vi "mainOcto_Scanning.vi"() -> ()   [LabVIEW 2013]
uses:
  <userlib>/Octoplus_LIDAR/GlobalNameAngles.vi
  <userlib>/Octoplus_LIDAR/Octoplus_LIDAR.lvlib
  <vilib>/Analysis/NI_AALBase.lvlib
panel:
  in  "start scan":bool
  in  "VISA resource name":refnum<visa-resource-name>
  in  "Time (ms)":u32
  in  "Azh":u16[](array[numeric])
  in  "Alt":u16[](array[numeric])
  in  "Nbr of lines in Image":u32=6000
  in  "File Path":path=path "D:/Sat25"
  in  "Capture":bool
  in  "Record data":bool
  in  "Timeslot (cw, ts1, ts2)":i32(knob)=2 scale=0.0..2.0
  out "Background":dbl[](graph)
  in  "start":bool
  out "Signal":dbl[][](graph)
  out "iteration":i32
  in  "stop":bool
  in  "error in (no error)":errorcluster
  out "error out":errorcluster
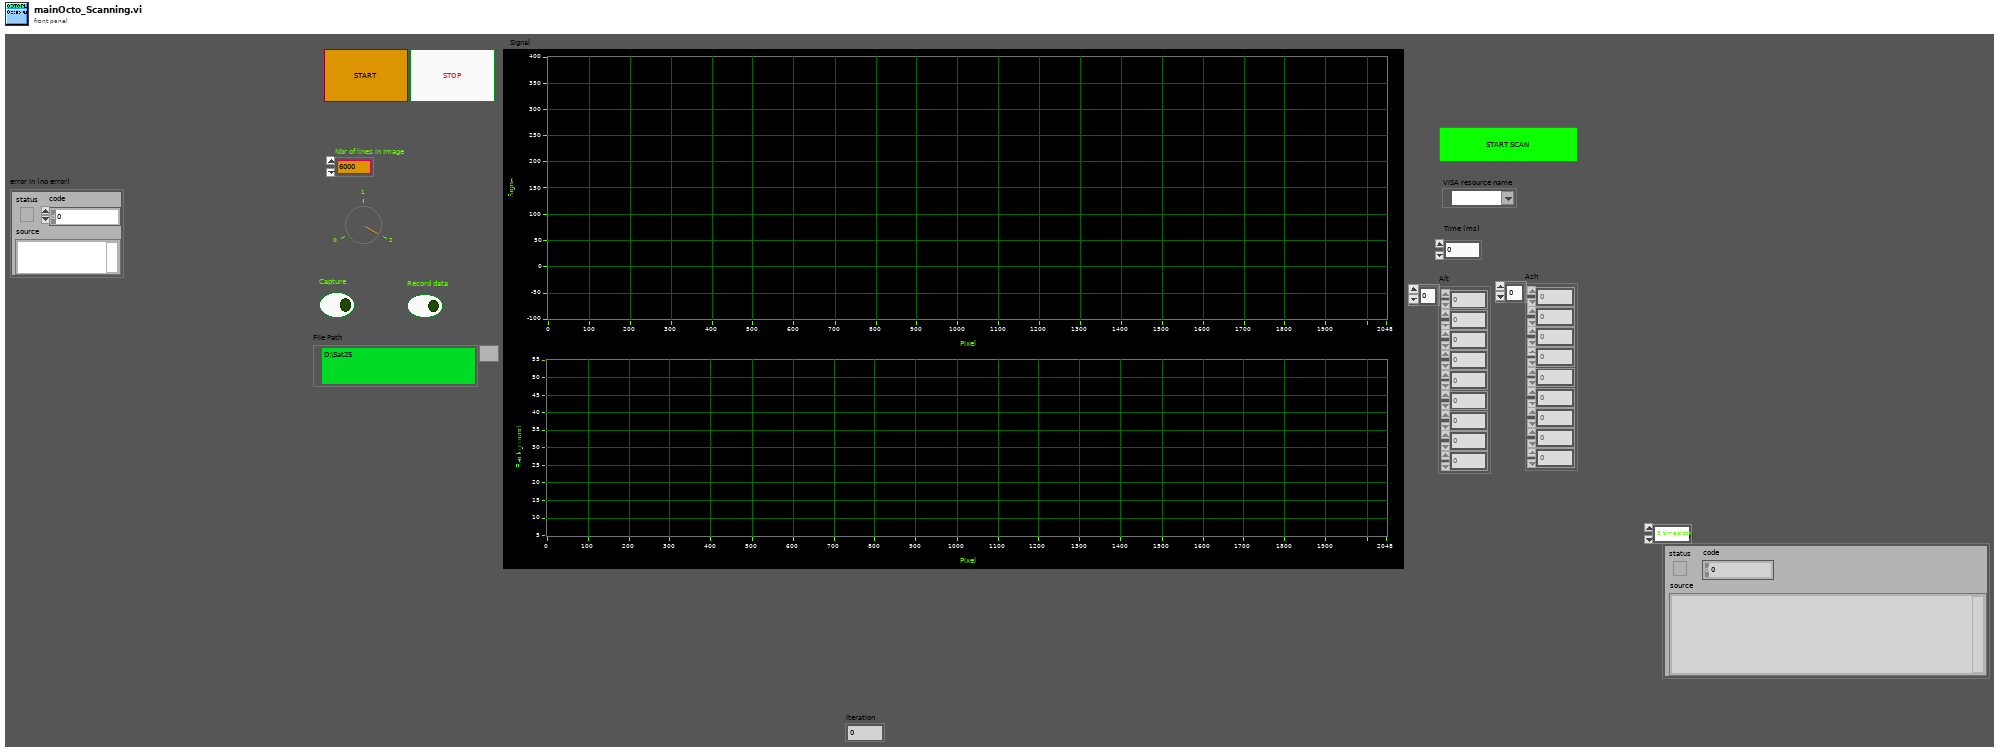
[diagram p1: front panel]
types:
  T1 = cluster{"pcID[0]":i8, "pcID[1]":i8, "pcID[2]":i8, "pcID[3]":i8, "pcID[4]":i8, "pcID[5]":i8, "pcID[6]":i8, "pcID[7]":i8, "pcID[8]":i8, "pcID[9]":i8, "pcID[10]":i8, "pcID[11]":i8, "pcID[12]":i8, "pcID[13]":i8, "pcID[14]":i8, "pcID[15]":i8, "pcID[16]":i8, "pcID[17]":i8, "pcID[18]":i8, "pcID[19]":i8, "pcID[20]":i8, "pcID[21]":i8, "pcID[22]":i8, "pcID[23]":i8, "pcID[24]":i8, "pcID[25]":i8, "pcID[26]":i8, "pcID[27]":i8, "pcID[28]":i8, "pcID[29]":i8, "pcID[30]":i8, "pcID[31]":i8, "pcID[32]":i8, "pcID[33]":i8, "pcID[34]":i8, "pcID[35]":i8, "pcID[36]":i8, "pcID[37]":i8, "pcID[38]":i8, "pcID[39]":i8, "pcID[40]":i8, "pcID[41]":i8, "pcID[42]":i8, "pcID[43]":i8, "pcID[44]":i8, "pcID[45]":i8, "pcID[46]":i8, "pcID[47]":i8, "pcID[48]":i8, "pcID[49]":i8, "pcID[50]":i8, "pcID[51]":i8, "pcID[52]":i8, "pcID[53]":i8, "pcID[54]":i8, "pcID[55]":i8, "pcID[56]":i8, "pcID[57]":i8, "pcID[58]":i8, "pcID[59]":i8, "pcID[60]":i8, "pcID[61]":i8, "pcID[62]":i8, "pcID[63]":i8, "pcID[64]":i8, "pcID[65]":i8, "pcID[66]":i8, "pcID[67]":i8, "pcID[68]":i8, "pcID[69]":i8, "pcID[70]":i8, "pcID[71]":i8, "pcID[72]":i8, "pcID[73]":i8, "pcID[74]":i8, "pcID[75]":i8, "pcID[76]":i8, "pcID[77]":i8, "pcID[78]":i8, "pcID[79]":i8, "pcID[80]":i8, "pcID[81]":i8, "pcID[82]":i8, "pcID[83]":i8, "pcID[84]":i8, "pcID[85]":i8, "pcID[86]":i8, "pcID[87]":i8, "pcID[88]":i8, "pcID[89]":i8, "pcID[90]":i8, "pcID[91]":i8, "pcID[92]":i8, "pcID[93]":i8, "pcID[94]":i8, "pcID[95]":i8, "pcID[96]":i8, "pcID[97]":i8, "pcID[98]":i8, "pcID[99]":i8, "pcID[100]":i8, "pcID[101]":i8, "pcID[102]":i8, "pcID[103]":i8, "pcID[104]":i8, "pcID[105]":i8, "pcID[106]":i8, "pcID[107]":i8, "pcID[108]":i8, "pcID[109]":i8, "pcID[110]":i8, "pcID[111]":i8, "pcID[112]":i8, "pcID[113]":i8, "pcID[114]":i8, "pcID[115]":i8, "pcID[116]":i8, "pcID[117]":i8, "pcID[118]":i8, "pcID[119]":i8, "pcID[120]":i8, "pcID[121]":i8, "pcID[122]":i8, "pcID[123]":i8, "pcID[124]":i8, "pcID[125]":i8, "pcID[126]":i8, "pcID[127]":i8, "pcID[128]":i8, "pcID[129]":i8, "pcID[130]":i8, "pcID[131]":i8, "pcID[132]":i8, "pcID[133]":i8, "pcID[134]":i8, "pcID[135]":i8, "pcID[136]":i8, "pcID[137]":i8, "pcID[138]":i8, "pcID[139]":i8, "pcID[140]":i8, "pcID[141]":i8, "pcID[142]":i8, "pcID[143]":i8, "pcID[144]":i8, "pcID[145]":i8, "pcID[146]":i8, "pcID[147]":i8, "pcID[148]":i8, "pcID[149]":i8, "pcID[150]":i8, "pcID[151]":i8, "pcID[152]":i8, "pcID[153]":i8, "pcID[154]":i8, "pcID[155]":i8, "pcID[156]":i8, "pcID[157]":i8, "pcID[158]":i8, "pcID[159]":i8, "pcID[160]":i8, "pcID[161]":i8, "pcID[162]":i8, "pcID[163]":i8, "pcID[164]":i8, "pcID[165]":i8, "pcID[166]":i8, "pcID[167]":i8, "pcID[168]":i8, "pcID[169]":i8, "pcID[170]":i8, "pcID[171]":i8, "pcID[172]":i8, "pcID[173]":i8, "pcID[174]":i8, "pcID[175]":i8, "pcID[176]":i8, "pcID[177]":i8, "pcID[178]":i8, "pcID[179]":i8, "pcID[180]":i8, "pcID[181]":i8, "pcID[182]":i8, "pcID[183]":i8, "pcID[184]":i8, "pcID[185]":i8, "pcID[186]":i8, "pcID[187]":i8, "pcID[188]":i8, "pcID[189]":i8, "pcID[190]":i8, "pcID[191]":i8, "pcID[192]":i8, "pcID[193]":i8, "pcID[194]":i8, "pcID[195]":i8, "pcID[196]":i8, "pcID[197]":i8, "pcID[198]":i8, "pcID[199]":i8, "pcID[200]":i8, "pcID[201]":i8, "pcID[202]":i8, "pcID[203]":i8, "pcID[204]":i8, "pcID[205]":i8, "pcID[206]":i8, "pcID[207]":i8, "pcID[208]":i8, "pcID[209]":i8, "pcID[210]":i8, "pcID[211]":i8, "pcID[212]":i8, "pcID[213]":i8, "pcID[214]":i8, "pcID[215]":i8, "pcID[216]":i8, "pcID[217]":i8, "pcID[218]":i8, "pcID[219]":i8, "pcID[220]":i8, "pcID[221]":i8, "pcID[222]":i8, "pcID[223]":i8, "pcID[224]":i8, "pcID[225]":i8, "pcID[226]":i8, "pcID[227]":i8, "pcID[228]":i8, "pcID[229]":i8, "pcID[230]":i8, "pcID[231]":i8, "pcID[232]":i8, "pcID[233]":i8, "pcID[234]":i8, "pcID[235]":i8, "pcID[236]":i8, "pcID[237]":i8, "pcID[238]":i8, "pcID[239]":i8, "pcID[240]":i8, "pcID[241]":i8, "pcID[242]":i8, "pcID[243]":i8, "pcID[244]":i8, "pcID[245]":i8, "pcID[246]":i8, "pcID[247]":i8, "pcID[248]":i8, "pcID[249]":i8, "pcID[250]":i8, "pcID[251]":i8, "pcID[252]":i8, "pcID[253]":i8, "pcID[254]":i8, "pcID[255]":i8, "pcID[256]":i8, "pcID[257]":i8, "pcID[258]":i8, "pcID[259]":i8}
  T2 = enum16{"open", "replace", "create", "open or create", "replace or create", "replace or create with confirmation"}
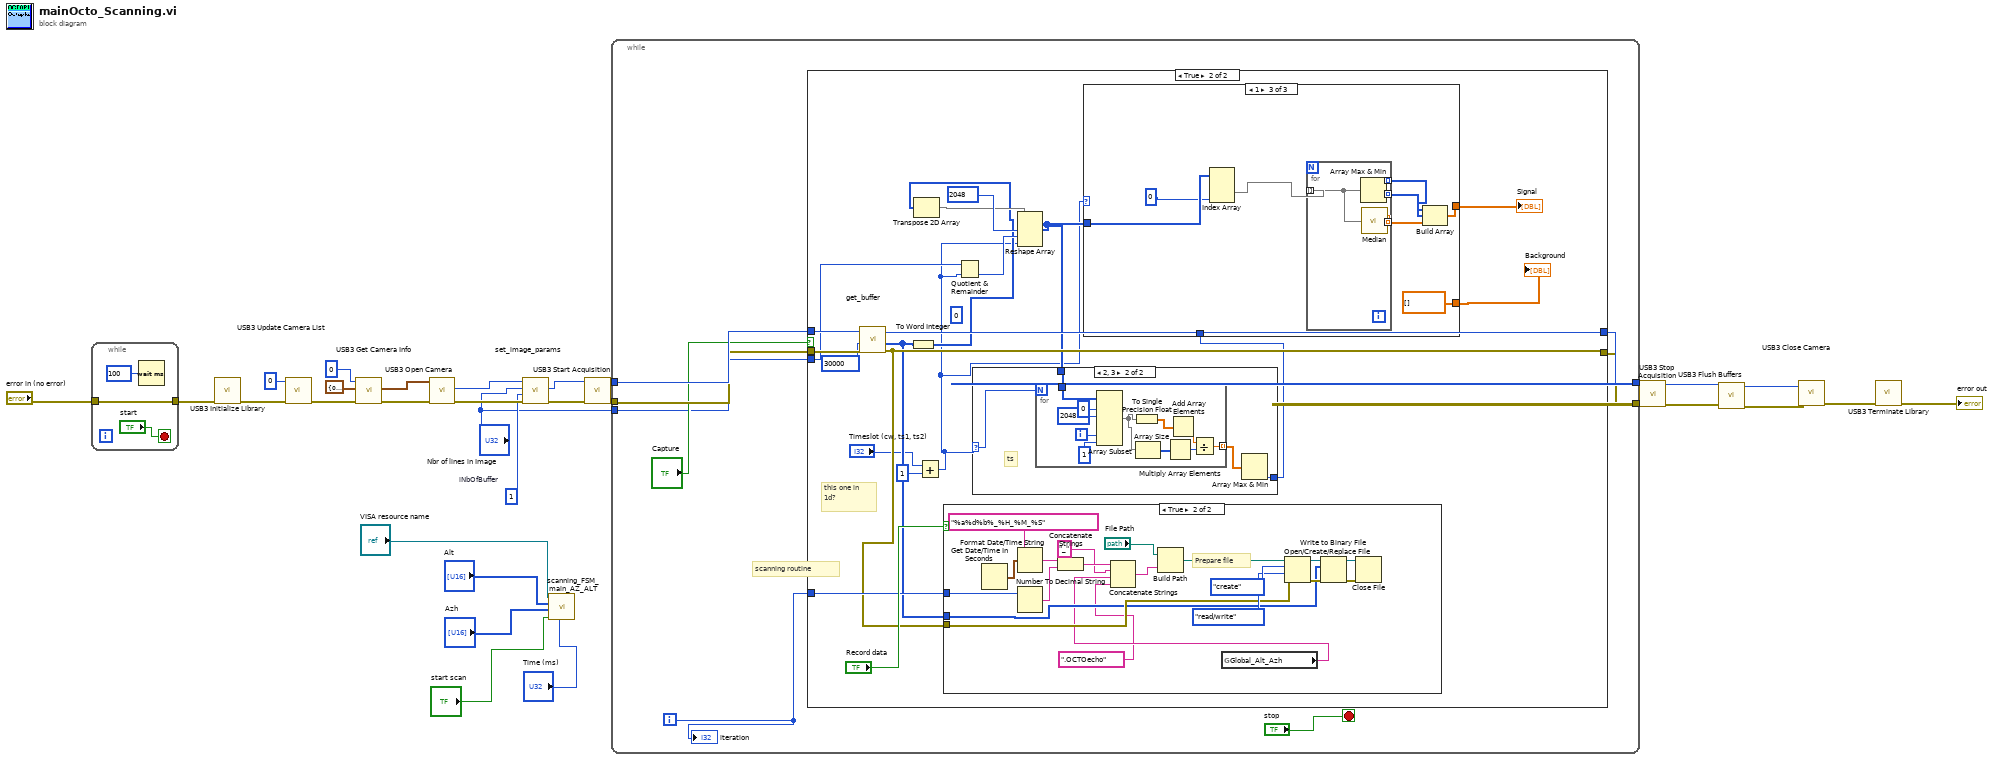
[diagram p0: block diagram]
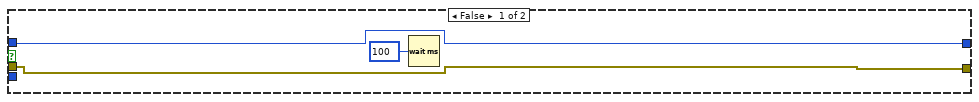
[diagram p2: hidden frame]
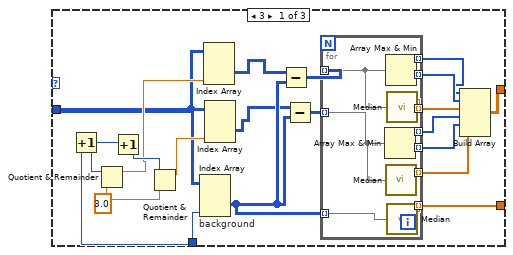
[diagram p3: hidden frame]
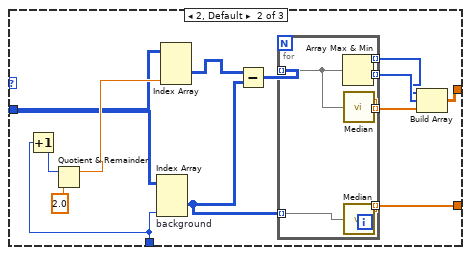
[diagram p4: hidden frame]
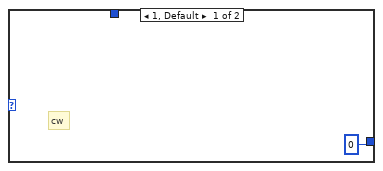
[diagram p6: hidden frame]
diagram:
  w22 = u32 1  # iNbOfBuffer
  n1 = while {
    tunnel: "error in (no error)" -> [w33]
    tunnel: [w33] -> w7
    stop <- "start" stop-if-true
    n2 = Wait (ms)(milliseconds to wait=u32 100) -> ()  [unwired: 1 out]
  }
  n3 = call <userlib>:"USB3 Initialize Library.vi"("error in (no error)"=w7) -> ("error out"=w9:errorcluster)  [unwired: 8 in, 1 out]
  n4 = call <userlib>:"USB3 Update Camera List.vi"("error in (no error)"=w9, "pulNbCameras"=u32 0) -> ("error out"=w27:errorcluster)  [unwired: 7 in, 2 out]
  n5 = call <userlib>:"USB3 Get Camera Info.vi"("error in (no error)"=w27, "pCameraInfo"=T1 {"pcID[0]"=0, "pcID[1]"=0, "pcID[2]"=0, "pcID[3]"=0, "pcID[4]"=0, "pcID[5]"=0, "pcID[6]"=0, "pcID[7]"=0, "pcID[8]"=0, "pcID[9]"=0, "pcID[10]"=0, "pcID[11]"=0, "pcID[12]"=0, "pcID[13]"=0, "pcID[14]"=0, "pcID[15]"=0, "pcID[16]"=0, "pcID[17]"=0, "pcID[18]"=0, "pcID[19]"=0, "pcID[20]"=0, "pcID[21]"=0, "pcID[22]"=0, "pcID[23]"=0, "pcID[24]"=0, "pcID[25]"=0, "pcID[26]"=0, "pcID[27]"=0, "pcID[28]"=0, "pcID[29]"=0, "pcID[30]"=0, "pcID[31]"=0, "pcID[32]"=0, "pcID[33]"=0, "pcID[34]"=0, "pcID[35]"=0, "pcID[36]"=0, "pcID[37]"=0, "pcID[38]"=0, "pcID[39]"=0, "pcID[40]"=0, "pcID[41]"=0, "pcID[42]"=0, "pcID[43]"=0, "pcID[44]"=0, "pcID[45]"=0, "pcID[46]"=0, "pcID[47]"=0, "pcID[48]"=0, "pcID[49]"=0, "pcID[50]"=0, "pcID[51]"=0, "pcID[52]"=0, "pcID[53]"=0, "pcID[54]"=0, "pcID[55]"=0, "pcID[56]"=0, "pcID[57]"=0, "pcID[58]"=0, "pcID[59]"=0, "pcID[60]"=0, "pcID[61]"=0, "pcID[62]"=0, "pcID[63]"=0, "pcID[64]"=0, "pcID[65]"=0, "pcID[66]"=0, "pcID[67]"=0, "pcID[68]"=0, "pcID[69]"=0, "pcID[70]"=0, "pcID[71]"=0, "pcID[72]"=0, "pcID[73]"=0, "pcID[74]"=0, "pcID[75]"=0, "pcID[76]"=0, "pcID[77]"=0, "pcID[78]"=0, "pcID[79]"=0, "pcID[80]"=0, "pcID[81]"=0, "pcID[82]"=0, "pcID[83]"=0, "pcID[84]"=0, "pcID[85]"=0, "pcID[86]"=0, "pcID[87]"=0, "pcID[88]"=0, "pcID[89]"=0, "pcID[90]"=0, "pcID[91]"=0, "pcID[92]"=0, "pcID[93]"=0, "pcID[94]"=0, "pcID[95]"=0, "pcID[96]"=0, "pcID[97]"=0, "pcID[98]"=0, "pcID[99]"=0, "pcID[100]"=0, "pcID[101]"=0, "pcID[102]"=0, "pcID[103]"=0, "pcID[104]"=0, "pcID[105]"=0, "pcID[106]"=0, "pcID[107]"=0, "pcID[108]"=0, "pcID[109]"=0, "pcID[110]"=0, "pcID[111]"=0, "pcID[112]"=0, "pcID[113]"=0, "pcID[114]"=0, "pcID[115]"=0, "pcID[116]"=0, "pcID[117]"=0, "pcID[118]"=0, "pcID[119]"=0, "pcID[120]"=0, "pcID[121]"=0, "pcID[122]"=0, "pcID[123]"=0, "pcID[124]"=0, "pcID[125]"=0, "pcID[126]"=0, "pcID[127]"=0, "pcID[128]"=0, "pcID[129]"=0, "pcID[130]"=0, "pcID[131]"=0, "pcID[132]"=0, "pcID[133]"=0, "pcID[134]"=0, "pcID[135]"=0, "pcID[136]"=0, "pcID[137]"=0, "pcID[138]"=0, "pcID[139]"=0, "pcID[140]"=0, "pcID[141]"=0, "pcID[142]"=0, "pcID[143]"=0, "pcID[144]"=0, "pcID[145]"=0, "pcID[146]"=0, "pcID[147]"=0, "pcID[148]"=0, "pcID[149]"=0, "pcID[150]"=0, "pcID[151]"=0, "pcID[152]"=0, "pcID[153]"=0, "pcID[154]"=0, "pcID[155]"=0, "pcID[156]"=0, "pcID[157]"=0, "pcID[158]"=0, "pcID[159]"=0, "pcID[160]"=0, "pcID[161]"=0, "pcID[162]"=0, "pcID[163]"=0, "pcID[164]"=0, "pcID[165]"=0, "pcID[166]"=0, "pcID[167]"=0, "pcID[168]"=0, "pcID[169]"=0, "pcID[170]"=0, "pcID[171]"=0, "pcID[172]"=0, "pcID[173]"=0, "pcID[174]"=0, "pcID[175]"=0, "pcID[176]"=0, "pcID[177]"=0, "pcID[178]"=0, "pcID[179]"=0, "pcID[180]"=0, "pcID[181]"=0, "pcID[182]"=0, "pcID[183]"=0, "pcID[184]"=0, "pcID[185]"=0, "pcID[186]"=0, "pcID[187]"=0, "pcID[188]"=0, "pcID[189]"=0, "pcID[190]"=0, "pcID[191]"=0, "pcID[192]"=0, "pcID[193]"=0, "pcID[194]"=0, "pcID[195]"=0, "pcID[196]"=0, "pcID[197]"=0, "pcID[198]"=0, "pcID[199]"=0, "pcID[200]"=0, "pcID[201]"=0, "pcID[202]"=0, "pcID[203]"=0, "pcID[204]"=0, "pcID[205]"=0, "pcID[206]"=0, "pcID[207]"=0, "pcID[208]"=0, "pcID[209]"=0, "pcID[210]"=0, "pcID[211]"=0, "pcID[212]"=0, "pcID[213]"=0, "pcID[214]"=0, "pcID[215]"=0, "pcID[216]"=0, "pcID[217]"=0, "pcID[218]"=0, "pcID[219]"=0, "pcID[220]"=0, "pcID[221]"=0, "pcID[222]"=0, "pcID[223]"=0, "pcID[224]"=0, "pcID[225]"=0, "pcID[226]"=0, "pcID[227]"=0, "pcID[228]"=0, "pcID[229]"=0, "pcID[230]"=0, "pcID[231]"=0, "pcID[232]"=0, "pcID[233]"=0, "pcID[234]"=0, "pcID[235]"=0, "pcID[236]"=0, "pcID[237]"=0, "pcID[238]"=0, "pcID[239]"=0, "pcID[240]"=0, "pcID[241]"=0, "pcID[242]"=0, "pcID[243]"=0, "pcID[244]"=0, "pcID[245]"=0, "pcID[246]"=0, "pcID[247]"=0, "pcID[248]"=0, "pcID[249]"=0, "pcID[250]"=0, "pcID[251]"=0, "pcID[252]"=0, "pcID[253]"=0, "pcID[254]"=0, "pcID[255]"=0, "pcID[256]"=0, "pcID[257]"=0, "pcID[258]"=0, "pcID[259]"=0}, "ulIndex"=u32 0) -> ("error out"=w25:errorcluster, "pCameraInfo out"=w26:T1)  [unwired: 6 in, 1 out]
  n6 = call <userlib>:"USB3 Open Camera.vi"("error in (no error)"=w25, "pCameraInfo"=w26) -> ("error out"=w24:errorcluster, "hCamera"=w23:u64)  [unwired: 7 in, 1 out]
  n7 = call <userlib>:"set_image_params.vi"("error in (no error)"=w24, "iNbOfBuffer"=w22, "iImageHeight"="Nbr of lines in Image", "hCamera"=w23) -> ("error out"=w21:errorcluster, "hCamera"=w12:u64)  [unwired: 5 in, 1 out]
  n8 = call <userlib>:"scanning_FSM_main_AZ_ALT.vi"("Time (ms)"="Time (ms)", "OK Button"="start scan", "AZH"="Azh", "ALT"="Alt", "VISA resource name"="VISA resource name") -> ()  [unwired: 5 in]
  n9 = call <userlib>:"USB3 Start Acquisition.vi"("error in (no error)"=w21, "hCamera"=w12) -> ("error out"=w19:errorcluster, "hCamera"=w20:u64)  [unwired: 7 in, 1 out]
  n10 = while {
    tunnel: w20 -> [w41]
    tunnel: w19 -> [w40]
    tunnel: [w37] -> w18
    tunnel: [w39] -> w15
    tunnel: "Nbr of lines in Image" -> [w35]
    i -> [w34]
    stop <- "stop" stop-if-true
    # "scanning routine"
    n11 = case shown="True" "Capture" {
      tunnel: w41 -> [w42 w64]
      tunnel: w40 -> [w43 w63]
      tunnel: [w42 w62] -> w39
      tunnel: [w43 w53] -> w37
      tunnel: w35 -> [_ w58]
      tunnel: w34 -> [_ w54]
      frame False {
        n12 = Wait (ms)(milliseconds to wait=u32 100) -> ()  [unwired: 1 out]
      }
      frame True {
        (unwired) 0 ("index")
        # "this one in\n1d?"
        n13 = call <userlib>:"get_buffer.vi"("error in (no error)"=w63, "ulTimeoutInMs"=u32 30000 ("Buffer timesout (ms)"), "hCamera"=w64) -> ("error out"=w53:errorcluster, "output array"=w48:u16[][], "hCamera out"=w62:u64)  [unwired: 5 in, 1 out]
        n14 = To Word Integer(number=w48) -> (16bit integer=w49:i16[][])
        n15 = Transpose 2D Array(2D array=w49) -> (transposed array=w50:i16[][])
        n16 = Add(x="Timeslot (cw, ts1, ts2)", y=1) -> (x+y=w45:i32)
        n17 = case shown="True" "Record data" {
          tunnel: w53 -> [_ w138]
          tunnel: w48 -> [_ w133]
          tunnel: w54 -> [_ w129]
          frame False {
          }
          frame True {
            # "Prepare file"
            n18 = Get Date/Time In Seconds() -> (seconds since 1Jan1904=w136:timestamp)
            n19 = Format Date/Time String(time format string (%c)="%a%d%b%_%H_%M_%S", seconds (now)=w136) -> (date/time string=w131:string)  [unwired: 1 in]
            n20 = Number To Decimal String(number=w129) -> (decimal integer string=w130:string)  [unwired: 1 in]
            n21 = Concatenate Strings(w131, w130) -> (w132:string)
            n22 = global read "GlobalNameAngles.vi" "Global_Alt_Azh"() -> (w127:string)
            n23 = Concatenate Strings(w132, "_", w127, ".OCTOecho") -> (w134:string)
            n24 = Build Path(base path="File Path", name or relative path=w134) -> (appended path=w137:path)
            n25 = Open/Create/Replace File(file path (use dialog)=w137, error in=w138, operation (0:open)=T2."create", access (0:read/write)=enum16{"read/write", "read-only", "write-only"}."read/write") -> (refnum out=w143:refnum<file>, error out=w139:errorcluster)  [unwired: 3 out]
            n26 = Write to Binary File(file (use dialog)=w143, data=w133, error in=w139) -> (refnum out=w141:refnum<file>, error out=w140:errorcluster)  [unwired: 1 in, 3 out]
            n27 = Close File(refnum=w141, error in=w140) -> ()  [unwired: 2 out]
          }
        }
        n28 = Quotient & Remainder(x=w58, y=w45) -> (floor(x/y)=w57:u32)  [unwired: 1 out]
        n29 = Reshape Array(w50, 2048 ("dimension size"), w57, w45) -> (w51:i16[][][])
        n30 = case shown="2, 3" w45 {
          selector: w45 -> [_ w147]
          tunnel: [0 w149] -> w52
          tunnel: w51 -> [_ w148]
          frame 1, Default {
            # "cw"
          }
          frame 2, 3 {
            # "ts"
            n31 = for {
              N: w147 -> [_]
              tunnel: [w160] -> w150 mode=indexing
              tunnel: w148 -> [w155]
              i -> [w157]
              n32 = Array Subset(array=w155, index (dim 0)=0 ("index"), length (dim 0)=2048 ("length"), index (dim 2)=w157, length (dim 2)=1 ("intervals")) -> (w152:i16[][][])  [unwired: 2 in]
              n33 = To Single Precision Float(number=w152) -> (single precision float=w151:sgl[][][])
              n34 = Array Size(array=w152) -> (size(s)=w158:i32[])
              n35 = Multiply Array Elements(1:w158) -> (0:w161:i32)
              n36 = Add Array Elements(numeric array=w151) -> (sum=w159:sgl)
              n37 = Divide(x=w159, y=w161) -> (x/y=w160:sgl)
            }
            n38 = Array Max & Min(array=w150) -> (min index (indices)=w149:i32)  [unwired: 3 out]
          }
        }
        n39 = case shown="1" w45 {
          tunnel: [w82 w105 dbl[] []] -> w60
          tunnel: [w81 w104 w119] -> w56
          tunnel: w52 -> [w76 w100 _]
          tunnel: w51 -> [w73 w98 w117]
          frame 3 {
            w78 = 3.0 ("y")
            n40 = Increment(x=w76) -> (x+1=w79:i32)
            n41 = Quotient & Remainder(x=w79, y=w78) -> (x-y*floor(x/y)=w75:dbl)  [unwired: 1 out]
            n42 = Increment(x=w79) -> (x+1=w77:i32)
            n43 = Quotient & Remainder(x=w77, y=w78) -> (x-y*floor(x/y)=w74:dbl)  [unwired: 1 out]
            n44 = Index Array "background"(array=w73, index (dim 2)=w76) -> (element=w72:i16[][])  [unwired: 2 in]
            n45 = Index Array(array=w73, index (dim 2)=w75) -> (element=w68:i16[][])  [unwired: 2 in]
            n46 = Index Array(array=w73, index (dim 2)=w74) -> (element=w71:i16[][])  [unwired: 2 in]
            n47 = Subtract(x=w68, y=w72) -> (x-y=w70:i16[][])
            n48 = Subtract(x=w71, y=w72) -> (x-y=w69:i16[][])
            n49 = for {
              tunnel: [w94] -> w80 mode=indexing
              tunnel: [w93] -> w84 mode=indexing
              tunnel: [w92] -> w83 mode=indexing
              tunnel: [w91] -> w82 mode=indexing
              tunnel: w72 -> [w90] mode=indexing
              tunnel: w70 -> [w89] mode=indexing
              tunnel: w69 -> [w88] mode=indexing
              tunnel: [w87] -> w67 mode=indexing
              tunnel: [w86] -> w66 mode=indexing
              tunnel: [w85] -> w65 mode=indexing
              n50 = Array Max & Min(array=w88) -> (max value=w87:i16, min value=w86:i16)  [unwired: 2 out]
              n51 = Array Max & Min(array=w89) -> (max value=w92:i16, min value=w93:i16)  [unwired: 2 out]
              n52 = call <vilib>:"Median.vi"("X"=w88) -> ("median"=w85:dbl)  [unwired: 1 out]
              n53 = call <vilib>:"Median.vi"("X"=w89) -> ("median"=w94:dbl)  [unwired: 1 out]
              n54 = call <vilib>:"Median.vi"("X"=w90) -> ("median"=w91:dbl)  [unwired: 1 out]
            }
            n55 = Build Array(w83, w84, w80, w67, w66, w65) -> (w81:dbl[][])
          }
          frame 2, Default {
            n56 = Increment(x=w100) -> (x+1=w102:i32)
            n57 = Quotient & Remainder(x=w102, y=2.0) -> (x-y*floor(x/y)=w99:dbl)  [unwired: 1 out]
            n58 = Index Array "background"(array=w98, index (dim 2)=w100) -> (element=w97:i16[][])  [unwired: 2 in]
            n59 = Index Array(array=w98, index (dim 2)=w99) -> (element=w95:i16[][])  [unwired: 2 in]
            n60 = Subtract(x=w95, y=w97) -> (x-y=w96:i16[][])
            n61 = for {
              tunnel: [w113] -> w103 mode=indexing
              tunnel: [w112] -> w107 mode=indexing
              tunnel: [w111] -> w106 mode=indexing
              tunnel: [w110] -> w105 mode=indexing
              tunnel: w97 -> [w109] mode=indexing
              tunnel: w96 -> [w108] mode=indexing
              n62 = Array Max & Min(array=w108) -> (max value=w111:i16, min value=w112:i16)  [unwired: 2 out]
              n63 = call <vilib>:"Median.vi"("X"=w108) -> ("median"=w113:dbl)  [unwired: 1 out]
              n64 = call <vilib>:"Median.vi"("X"=w109) -> ("median"=w110:dbl)  [unwired: 1 out]
            }
            n65 = Build Array(w106, w107, w103) -> (w104:dbl[][])
          }
          frame 1 {
            n66 = Index Array(array=w117, index (dim 2)=0 ("index (col)")) -> (element=w115:i16[][])  [unwired: 2 in]
            n67 = for {
              tunnel: [w125] -> w118 mode=indexing
              tunnel: [w124] -> w121 mode=indexing
              tunnel: [w123] -> w120 mode=indexing
              tunnel: w115 -> [w122] mode=indexing
              n68 = Array Max & Min(array=w122) -> (max value=w123:i16, min value=w124:i16)  [unwired: 2 out]
              n69 = call <vilib>:"Median.vi"("X"=w122) -> ("median"=w125:dbl)  [unwired: 1 out]
            }
            n70 = Build Array(w120, w121, w118) -> (w119:dbl[][])
          }
        }
        "Signal" <- w56
        "Background" <- w60
      }
    }
    "iteration" <- w34
  }
  n71 = call <userlib>:"USB3 Stop Acquisition.vi"("error in (no error)"=w18, "hCamera"=w15) -> ("error out"=w17:errorcluster, "hCamera out"=w14:u64)  [unwired: 7 in, 1 out]
  n72 = call <userlib>:"USB3 Flush Buffers.vi"("error in (no error)"=w17, "hCamera"=w14) -> ("error out"=w16:errorcluster, "hCamera out"=w13:u64)  [unwired: 7 in, 1 out]
  n73 = call <userlib>:"USB3 Close Camera.vi"("error in (no error)"=w16, "hCamera"=w13) -> ("error out"=w11:errorcluster)  [unwired: 7 in, 2 out]
  n74 = call <userlib>:"USB3 Terminate Library.vi"("error in (no error)"=w11) -> ("error out"=→"error out":errorcluster)  [unwired: 9 in, 1 out]
